vi "ep_Append Data.vi"(0 "history data":dbl[][](array[numeric]), 5 "current data":dbl[][](array[numeric]), 9 "system info in":refnum<class "EP System Info.lvclass">, 11 "error in (no error)":errorcluster) -> (4 "appended signal":dbl[][](array[numeric]), 6 "total cycles":i32, 8 "total size":i32, 10 "system info out":refnum<class "EP System Info.lvclass">, 15 "error out":errorcluster)   [LabVIEW 2013, in "NI_EP_Power Quality.lvlib"]
uses:
  <vilib>/addons/Electrical Power/PQ/Common/Classes/System Info/EP System Info.lvclass
  <vilib>/addons/Electrical Power/PQ/NI_EP_Power Quality.lvlib
  <vilib>/addons/Electrical Power/Power Measurement/NI_EP_Power Measurement.lvlib
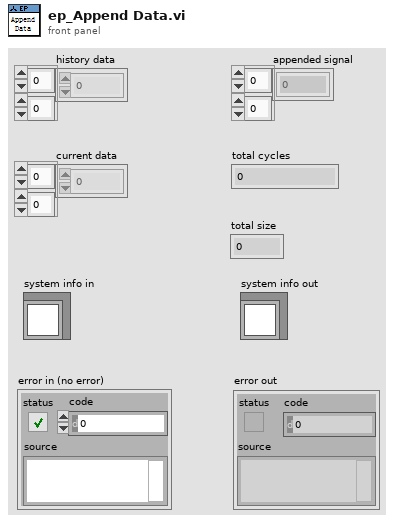
[diagram p1: front panel]
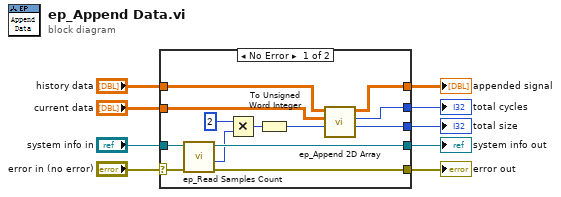
[diagram p0: block diagram]
diagram:
  n1 = case shown="No Error" "error in (no error)" {
    selector: "error in (no error)" -> [w17 w24]
    tunnel: "current data" -> [w13 _]
    tunnel: [w14 _] -> w8
    tunnel: [w10 _] -> w7
    tunnel: "history data" -> [w12 _]
    tunnel: [w11 _] -> w5
    tunnel: "system info in" -> [w22 w23]
    tunnel: [w21 w23] -> w3
    tunnel: [w20 w24] -> w2
    frame No Error {
      n2 = call <vilib>:"ep_Read Samples Count.vi"("error in (no error)"=w17, "system info in"=w22) -> ("error out"=w20:errorcluster, "half-cycle (samples)"=w19:i32, "system info out"=w21:refnum<class "EP System Info.lvclass">)  [unwired: 5 in, 2 out]
      n3 = Multiply(x=2, y=w19) -> (x*y=w16:i32)
      n4 = To Unsigned Word Integer(number=w16) -> (unsigned 16bit integer=w15:u16)
      n5 = call <vilib>:"ep_Append 2D Array.vi"("samples per cycle"=w15, "current data"=w13, "history data"=w12) -> ("total size"=w11:i32, "total cycles"=w10:i32, "appended data"=w14:dbl[][])  [unwired: 6 in]
    }
    frame Error {
    }
  }
  "appended signal" <- w8
  "system info out" <- w3
  "total cycles" <- w7
  "total size" <- w5
  "error out" <- w2
